vi "D_bank_Manual_Control_02.vi"(0 "SI804.lvclass in":refnum<class "SI804.lvclass">, 1 "3 JSD20 DT302\nXA01":bool, 2 "3 JSD20 DT301\nXA01":bool, 3 "3 JSD20 DT303\nXA01":bool, 5 "error in":errorcluster) -> (14 "SI804.lvclass out":refnum<class "SI804.lvclass">, 15 "D-Bank ins":bool, 16 "L-bank Ctrl M/A":bool, 17 "D-bank withdr":bool, 19 "error out":errorcluster)   [LabVIEW 2022 SP3, in "SI804.lvclass"]
uses:
  SI804.lvclass
  SI804.lvclass/SI804.ctl
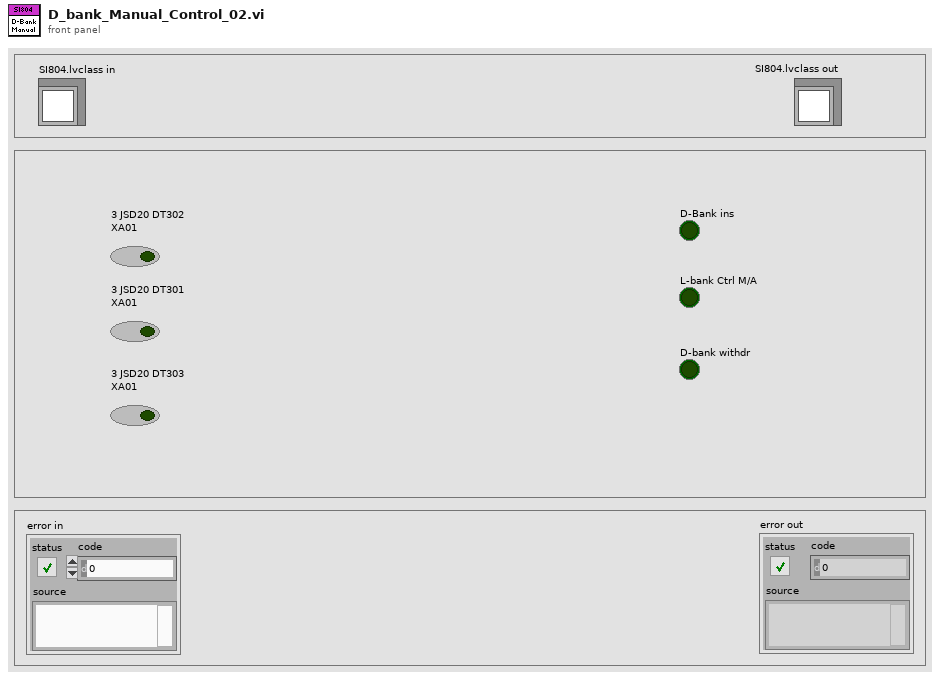
[diagram p1: front panel]
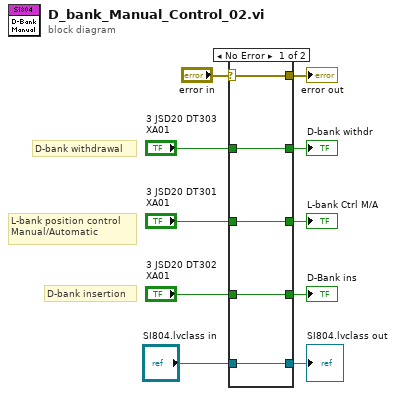
[diagram p0: block diagram]
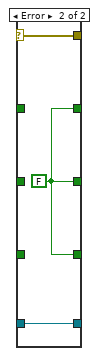
[diagram p2: hidden frame]
diagram:
  # "D-bank withdrawal"
  # "L-bank position control\nManual/Automatic"
  # "D-bank insertion"
  n1 = case shown="No Error" "error in" {
    selector: "error in" -> [w12 w17]
    tunnel: "3 JSD20 DT302\nXA01" -> [w15 _]
    tunnel: "3 JSD20 DT301\nXA01" -> [w14 _]
    tunnel: "3 JSD20 DT303\nXA01" -> [w13 _]
    tunnel: [w15 w18] -> w6
    tunnel: [w14 w18] -> w5
    tunnel: [w13 w18] -> w4
    tunnel: [w12 w17] -> w3
    tunnel: "SI804.lvclass in" -> [w11 w16]
    tunnel: [w11 w16] -> w1
    frame No Error {
    }
    frame Error {
      w18 = FALSE ("3 JSD20 DT302\nXA01")
    }
  }
  "D-Bank ins" <- w6
  "L-bank Ctrl M/A" <- w5
  "D-bank withdr" <- w4
  "error out" <- w3
  "SI804.lvclass out" <- w1
